vi "Translate_TREECONTROL.vi"(8 "error IN":errorcluster, 10 "Cle":string, 11 "Tree Refnum":refnum<vi>) -> (0 "error out":errorcluster)   [LabVIEW 2013]
uses:
  Dictionnary/EnumCommandDictionnaire.ctl
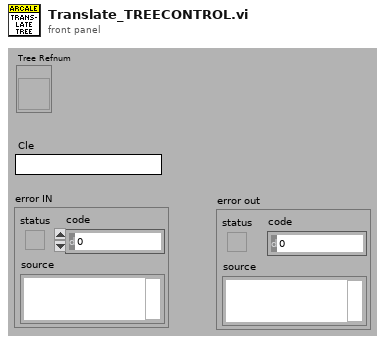
[diagram p1: front panel]
types:
  T1 = typedef "EnumCommandDictionnaire.ctl" = enum16{"Load", "Translate", "Save", "GetDico", "Set : A traduire = Vrai", "Set : A Traduire = Faux", "SetDico"}
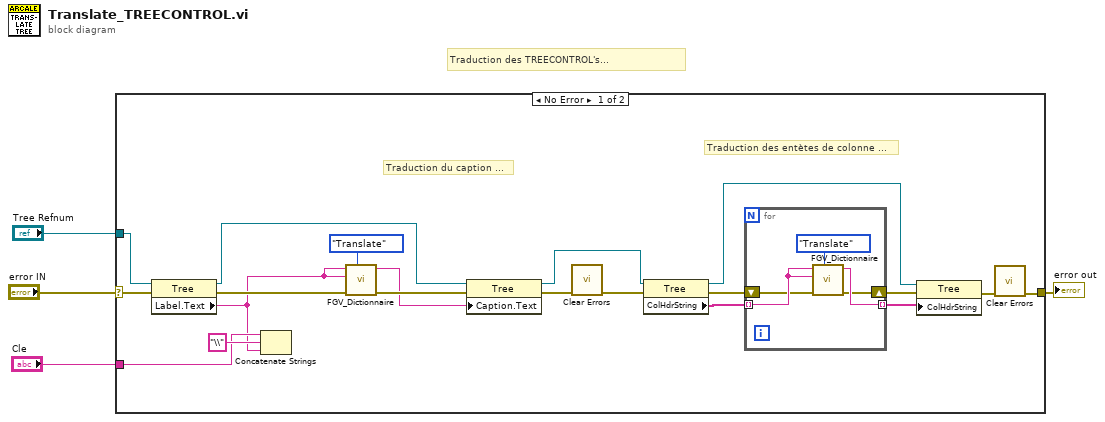
[diagram p0: block diagram]
diagram:
  # "Traduction des TREECONTROL's..."
  n1 = case shown="No Error" "error IN" {
    selector: "error IN" -> [w24 w30]
    tunnel: "Tree Refnum" -> [w23 _]
    tunnel: "Cle" -> [w19 _]
    tunnel: [w8 w30] -> w1
    frame No Error {
      # "Traduction des entètes de colonne ..."
      # "Traduction du caption ..."
      n2 = property class="Tree"(reference=w23, error in=w24) -> (reference out=w20:refnum<vi>, error out=w17:errorcluster, "Label.Text"=w14:string)
      n3 = Concatenate Strings(w19, "\\" ("string"), w14) -> ()  [unwired: 1 out]
      n4 = call "FGV_Dictionnaire.vi"("Command"=EnumCommandDictionnaire."Translate", "error in (no error)"=w17, "Chaîne"=w14, "Clé"=w14) -> ("error out"=w16:errorcluster, "Traduction"=w15:string)  [unwired: 5 in, 1 out]
      n5 = property class="Tree"(reference=w20, error in=w16, "Caption.Text"=w15) -> (reference out=w12:refnum<vi>, error out=w21:errorcluster)
      n6 = call <vilib>:"Clear Errors.vi"("error in (no error)"=w21) -> ("error out"=w13:errorcluster)  [unwired: 6 in]
      n7 = property class="Tree"(reference=w12, error in=w13) -> (reference out=w6:refnum<vi>, error out=w10:errorcluster, "ColHdrString"=w11:string[])
      n8 = for {
        tunnel: w11 -> [w29] mode=indexing
        tunnel: [w27] -> w7 mode=indexing
        shift-right: [w25] -> w5
        shift-left: w10 -> [w28]
        n9 = call "FGV_Dictionnaire.vi"("Command"=EnumCommandDictionnaire."Translate", "error in (no error)"=w28, "Chaîne"=w29, "Clé"=w29) -> ("error out"=w25:errorcluster, "Traduction"=w27:string)  [unwired: 5 in, 1 out]
      }
      n10 = property class="Tree"(reference=w6, error in=w5, "ColHdrString"=w7) -> (error out=w9:errorcluster)  [unwired: 1 out]
      n11 = call <vilib>:"Clear Errors.vi"("error in (no error)"=w9) -> ("error out"=w8:errorcluster)  [unwired: 6 in]
    }
    frame Error {
    }
  }
  "error out" <- w1
